vi "Read TopRow.vi"(8 "error in (no error)":errorcluster, 11 "BetterListboxHandle in":refnum<class "BetterListboxHandle.lvclass">) -> (0 "error out":errorcluster, 2 "Top Row":i32, 3 "BetterListboxHandle out":refnum<class "BetterListboxHandle.lvclass">)   [LabVIEW 2020, in "BetterDragAndDrop.lvlib" / "BetterListboxHandle.lvclass"]
uses:
  BetterListboxHandle.lvclass
  BetterListboxHandle.lvclass/BetterListboxHandle.ctl
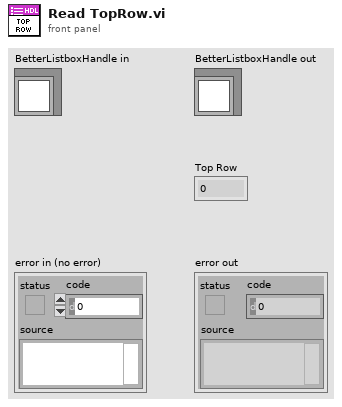
[diagram p1: front panel]
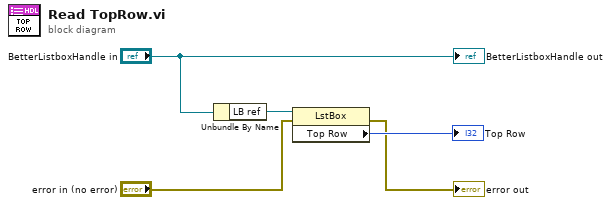
[diagram p0: block diagram]
diagram:
  n1 = Unbundle By Name("BetterListboxHandle in") -> ("LB ref"=w4:refnum<vi>)
  n2 = property class="LstBox"(reference=w4, error in="error in (no error)") -> (error out=→"error out":errorcluster, "Top Row"=→"Top Row":i32)  [unwired: 1 out]
  "BetterListboxHandle out" <- "BetterListboxHandle in"
